vi "Test Connection.vi"(8 "error in (no error)":errorcluster, 11 "TCP Network Connection in":refnum<k5>) -> (0 "error out":errorcluster, 2 "Model type":string, 3 "TCP Network Connection out":refnum<k5>)   [LabVIEW 2019, in "FX5U SLMP Binary.lvlib"]
uses:
  FX5U SLMP Binary.lvlib
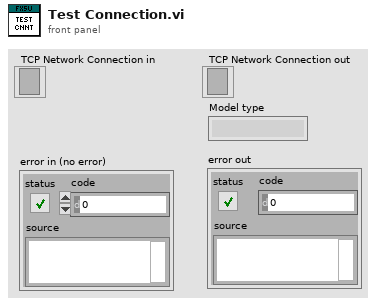
[diagram p1: front panel]
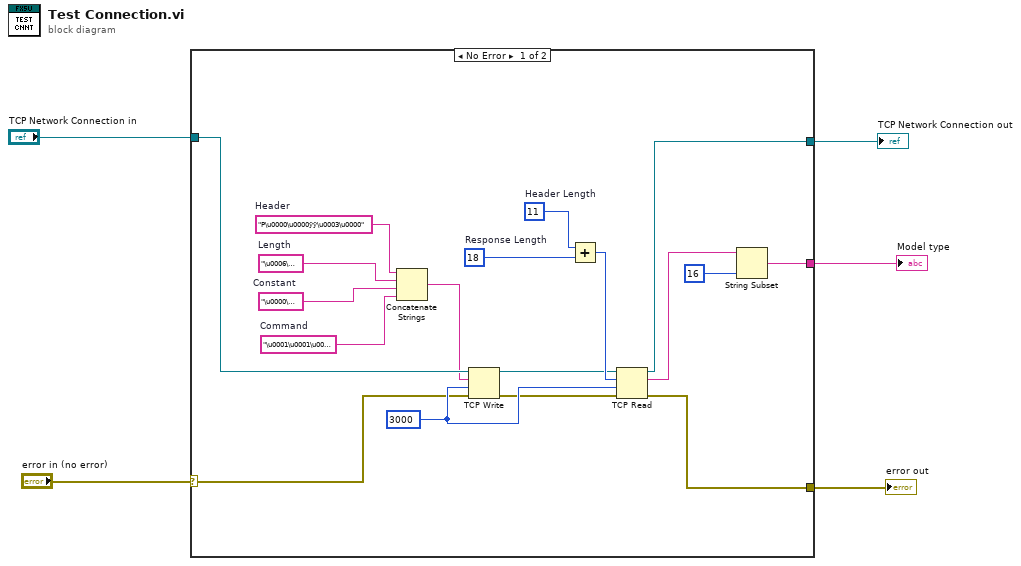
[diagram p0: block diagram]
diagram:
  n1 = case shown="No Error" "error in (no error)" {
    selector: "error in (no error)" -> [w6 w24]
    tunnel: [w23 w25] -> w5
    tunnel: [w22 w24] -> w4
    tunnel: "TCP Network Connection in" -> [w21 w25]
    tunnel: [w8 _] -> w2
    frame No Error {
      w18 = 18  # Response Length
      w19 = 11  # Header Length
      w17 = 3000 ("timeout ms (25000)")
      w16 = "\u0001\u0001\u0000\u0000"  # Command
      w15 = "\u0000\u0000"  # Constant
      w14 = "\u0006\u0000"  # Length
      w13 = "P\u0000\u0000ÿÿ\u0003\u0000"  # Header
      n2 = Concatenate Strings(w13, w14, w15, w16) -> (w12:string)
      n3 = TCP Write(connection ID=w21, data in=w12, error in (no error)=w6, 9:w17) -> (connection ID out=w10:refnum<k5>, error out=w11:errorcluster)  [unwired: 1 out]
      n4 = Add(x=w19, y=w18) -> (x+y=w20:i32)
      n5 = TCP Read(connection ID=w10, bytes to read=w20, error in (no error)=w11, 9:w17) -> (connection ID out=w23:refnum<k5>, data out=w7:string, error out=w22:errorcluster)  [unwired: 1 in]
      n6 = String Subset(string=w7, length (rest)=16 ("length (rest)")) -> (substring=w8:string)  [unwired: 1 in]
    }
    frame Error {
    }
  }
  "TCP Network Connection out" <- w5
  "error out" <- w4
  "Model type" <- w2
